vi "Global Monitor.vi"() -> ()   [LabVIEW 2018, in "VICI M6 M50 Party Mode.lvlib" / "VICI Global Library.lvlib"]
uses:
  VICI Global Library.lvlib
  VICI Global Array.ctl
  VICI Global.ctl
panel:
  in  "Wipe Global":bool
  out "VICI Pump Global":T1
  in  "stop":bool
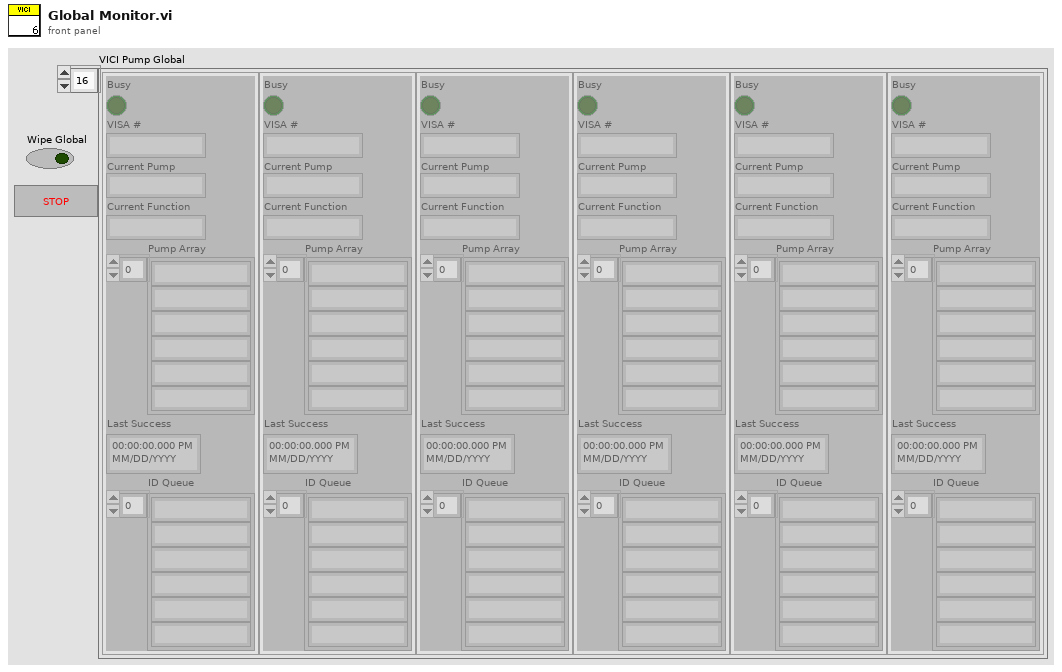
[diagram p1: front panel]
types:
  T1 = typedef "VICI M6 M50 Party Mode.lvlib/VICI Global Library.lvlib/VICI Global Array.ctl" = T2[]
  T2 = typedef "VICI M6 M50 Party Mode.lvlib/VICI Global Library.lvlib/VICI Global.ctl" = cluster{"Busy":bool, "VISA #":string, "Current Pump":string, "Current Function":string, "Pump Array":string[], "Last Success":timestamp, "ID Queue":string[]}
  T3 = cluster{"Busy":bool, "VISA #":string, "Current Pump":string, "Current Function":string, "Pump Array":string[], "Last Success":timestamp, "ID Queue":string[]}[]
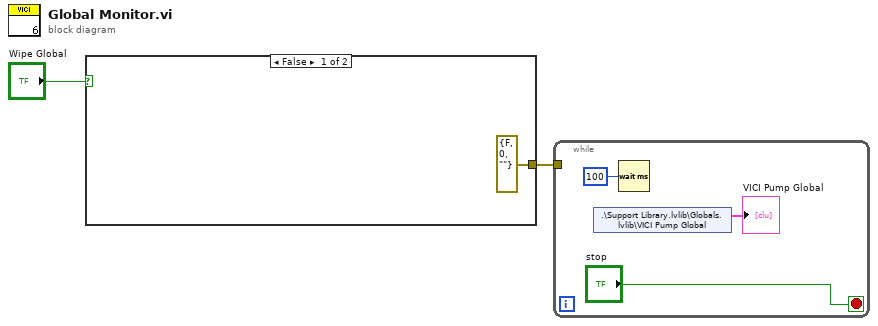
[diagram p0: block diagram]
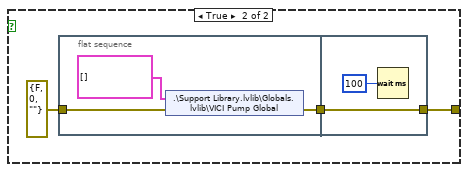
[diagram p2: hidden frame]
diagram:
  n1 = case shown="False" "Wipe Global" {
    tunnel: [errorcluster {"status"=FALSE, "code"=0, "source"=""} ("error IO") w5] -> w2
    frame False {
    }
    frame True {
      n2 = flat-sequence {
        tunnel: [w9] -> w6
        tunnel: errorcluster {"status"=FALSE, "code"=0, "source"=""} ("error in (no error)") -> [w8]
        tunnel: w6 -> [w11]
        tunnel: [w11] -> w5
        frame #0 {
          n3 = shared-variable ".\\Support Library.lvlib\\Globals.lvlib\\VICI Pump Global"(T1 [] ("VICI Pump Global"), error in=w8) -> (error out=w9:errorcluster)
        }
        frame #1 {
          n4 = Wait (ms)(milliseconds to wait=u32 100) -> ()  [unwired: 1 out]
        }
      }
    }
  }
  n5 = while {
    tunnel: w2 -> [_]
    stop <- "stop" stop-if-true
    n6 = shared-variable ".\\Support Library.lvlib\\Globals.lvlib\\VICI Pump Global"() -> (→"VICI Pump Global":T3)  [unwired: 1 in, 1 out]
    n7 = Wait (ms)(milliseconds to wait=u32 100) -> ()  [unwired: 1 out]
  }
